vi "set_iterations_per_pixel.vi"(8 "error in (no error)":errorcluster, 10 "iterations per pixel":i32, 11 "FPGAWrapperDL090211Galvo in":refnum<class "FPGAWrapperDL090211Galvo_grabber.lvclass">) -> (0 "error out":errorcluster, 3 "FPGAWrapperDL090211Galvo out":refnum<class "FPGAWrapperDL090211Galvo_grabber.lvclass">)   [LabVIEW 2010, in "FPGAWrapperDL090211Galvo_grabber.lvclass"]
uses:
  FPGAWrapperDL090211Galvo_grabber.lvclass
  FPGAWrapperDL090211Galvo_grabber.lvclass/FPGAWrapperDL090211Galvo_grabber.ctl
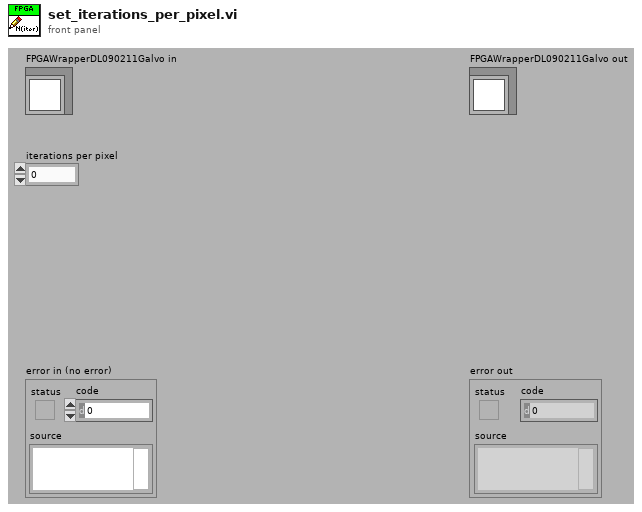
[diagram p1: front panel]
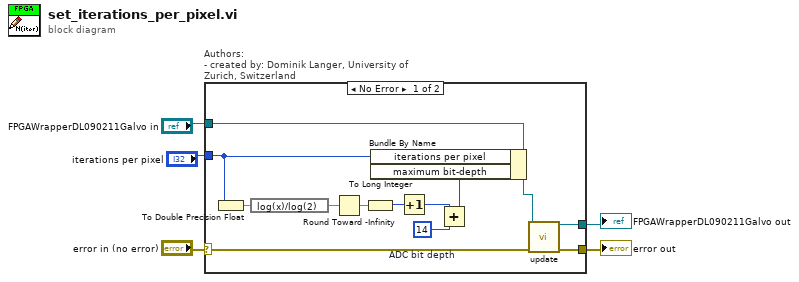
[diagram p0: block diagram]
diagram:
  n1 = case "Authors: \n- created by: Dominik Langer, University of Zurich, Switzerland" shown="No Error" "error in (no error)" {
    selector: "error in (no error)" -> [w9 w19]
    tunnel: "FPGAWrapperDL090211Galvo in" -> [w12 w20]
    tunnel: [w7 w20] -> w1
    tunnel: [w6 w19] -> w2
    tunnel: "iterations per pixel" -> [w11 _]
    frame No Error {
      w17 = 14  # ADC bit depth
      n2 = To Double Precision Float(number=w11) -> (double precision float=w14:dbl)
      n3 = expression code="log(x)/log(2)"(w14) -> (w13:dbl)
      n4 = Round Toward -Infinity(1:w13) -> (0:w18:dbl)
      n5 = To Long Integer(number=w18) -> (32bit integer=w16:i32)
      n6 = Increment(x=w16) -> (x+1=w15:i32)
      n7 = Add(x=w15, y=w17) -> (x+y=w10:i32)
      n8 = Bundle By Name(cluster=w12, "iterations per pixel"=w11, "maximum bit-depth"=w10) -> (w8:refnum<class "FPGAWrapperDL090211Galvo_grabber.lvclass">)
      n9 = call-dynamic "update.vi"("error in (no error)"=w9, "FPGAWrapperDL120115Galvo in"=w8) -> ("error out"=w6:errorcluster, "FPGAWrapperDL120115Galvo out"=w7:refnum<class "FPGAWrapperDL090211Galvo_grabber.lvclass">)  [unwired: 8 in]
    }
    frame Error {
    }
  }
  "error out" <- w2
  "FPGAWrapperDL090211Galvo out" <- w1
